vi "Set settings chain.vi"(8 "error in (no error)":errorcluster, 9 "class name":string[](array[string]), 10 "settings":variant[](array[variant]), 11 "Template in":refnum<class "Template.lvclass">) -> (0 "error out":errorcluster, 3 "Template out":refnum<class "Template.lvclass">)   [LabVIEW 2012, in "Template.lvclass"]
uses:
  Template.lvclass
  <vilib>/Distrio/Murmex/Murmex/Murmex.lvclass
  Template.lvclass/Template.ctl
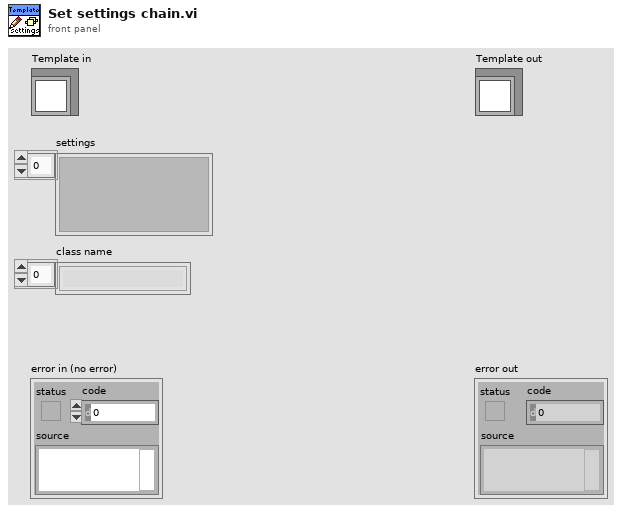
[diagram p1: front panel]
types:
  T1 = typedef "Template.lvclass/settings_cluster.ctl" = cluster{"frequency":dbl}
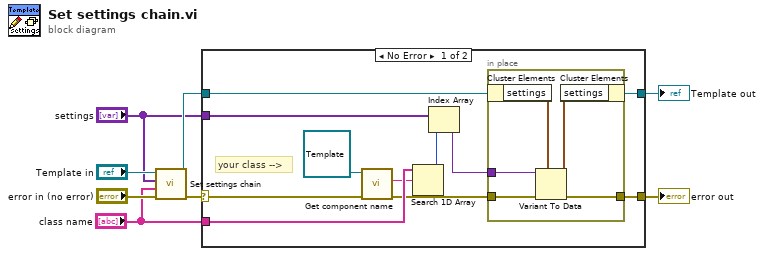
[diagram p0: block diagram]
diagram:
  n1 = call-parent "Set settings chain.vi"("error in (no error)"="error in (no error)", "class name"="class name", "settings"="settings", "Murmex in"="Template in") -> ("error out"=w5:errorcluster, "Murmex out"=w6:refnum<class "Template.lvclass">)  [unwired: 6 in]
  n2 = case shown="No Error" w5 {
    selector: w5 -> [w19 w26]
    tunnel: [w10 w26] -> w4
    tunnel: [w11 w25] -> w3
    tunnel: w6 -> [w12 w25]
    tunnel: "class name" -> [w18 _]
    tunnel: "settings" -> [w16 _]
    frame No Error {
      # "your class -->"
      n3 = call <vilib>:"Get component name.vi"("error in (no error)"=w19, "Murmex in"=refnum<class "Template.lvclass"> refnum ("Murmex out")) -> ("error out"=w13:errorcluster, "component name"=w17:string)  [unwired: 7 in, 1 out]
      n4 = Search 1D Array(1D array=w18, element=w17) -> (index of element=w15:i32)  [unwired: 1 in]
      n5 = Index Array(array=w16, index=w15) -> (element=w14:variant)
      n6 = in-place {
        in-place-border: w14 -> [w24]
        in-place-border: w13 -> [w22]
        in-place-border: [w20] -> w10
        n7 = in-place-cluster #1(w12) -> ("settings"=w23:T1)
        n8 = Variant To Data(error in=w22, type=w23, Variant=w24) -> (data=w21:T1, error out=w20:errorcluster)
        n9 = in-place-cluster #1("settings"=w21) -> (w11:refnum<class "Template.lvclass">)
      }
    }
    frame Error {
    }
  }
  "error out" <- w4
  "Template out" <- w3
